vi "CSM - Run Script.vi"(0 "CSM Scripts":string, 1 "Current Module (\"\" to Generate an ID)":string, 7 "Continue If Error? (F)":bool, 9 "Wait (5000ms)":i32=5000, 11 "error in (no error)":errorcluster, 12 "Response Timeout (-2 Using Global Settings)":i32=-2) -> (4 "Response":string[](array[string]), 10 "Scripts Left":string, 15 "error out":errorcluster)   [LabVIEW 2017, in "Communicable State Machine.lvlib"]
doc: "Executes multiple CSM commands in a single batch, supporting synchronous messages, asynchronous messages, and subscriptions.\n\n\n> [!NOTE] <b>CSM Message Target Module Description</b>\n>\n> In Normal Mode, the target module for a CSM message is the specified module name. System-level modules start with a `.` in their name. The target module for a CSM message includes the `.` in the name. For example, if the requested module name is `.System`, the target module for the CSM message is `.System`. In Worker Mode, the target module for a CSM message can only be the overall module name, not the node name. For example, if the requested module name is `Worker#`, the target module for the CSM message is `Worker`. In Chain of Responsibility Mode, the target module for a CSM message can only be the overall module name, not the node name. For example, if the requested module name is `Chain$1`, the target module for the CSM message is `Chain`.\n\n\n-- <b>Controls</b> --\n- <b>Current Module (\"\" to Generate an ID)</b>: Name of the current module. If empty, a temporary ID is generated for debugging purposes to identify the location.\n- <b>CSM Scripts</b>: CSM commands to execute.\n- <b>Continue If Error? (F)</b>: Whether to continue execution if an error occurs. The default is FALSE, which specifies to not continue.\n- <b>Wait (5000 ms)</b>: Timeout duration for waiting. The default is 5000 ms.\n- <b>Response Timeout (-2 Using Global Settings)</b>: Timeout for synchronous calls. The default is -2, which uses the global setting. You can set the global timeout using the CSM - Set TMO of Sync-Reply VI.\n\n-- <b>Indicators</b> --\n- <b>Response</b>: Returned results from executing the script. Only synchronous messages carry returns. The corresponding column for other commands will be an empty string.\n- <b>Scripts Left</b>: Remaining unexecuted scripts."
uses:
  Communicable State Machine.lvlib
  _Shared/CSM Shared.lvlib
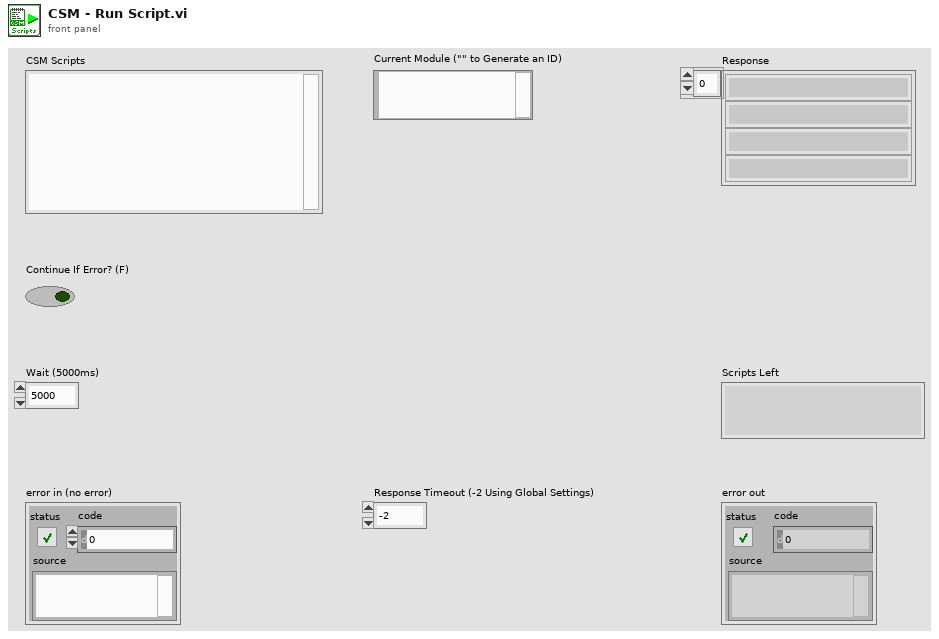
[diagram p1: front panel]
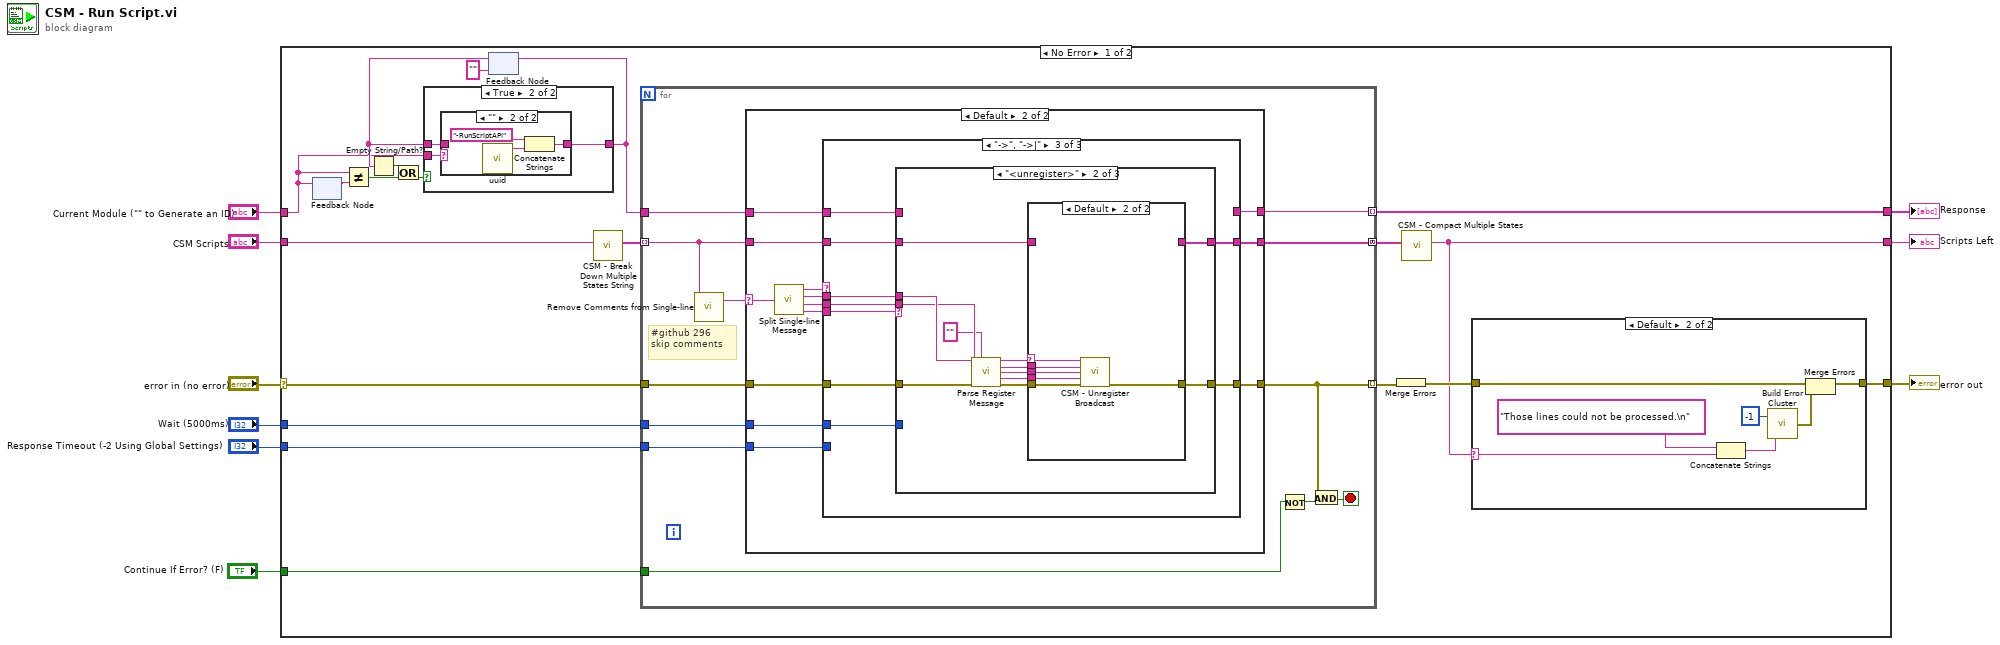
[diagram p0: block diagram]
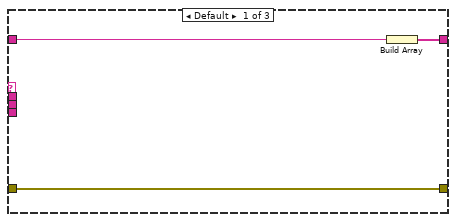
[diagram p6: hidden frame]
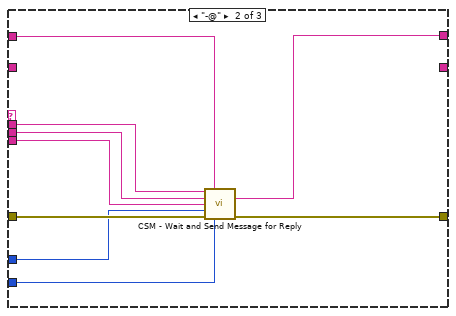
[diagram p7: hidden frame]
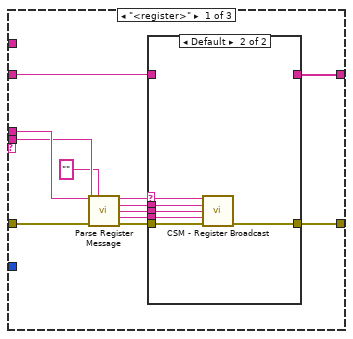
[diagram p8: hidden frame]
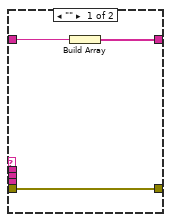
[diagram p9: hidden frame]
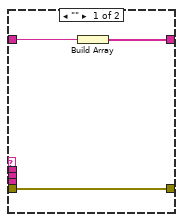
[diagram p10: hidden frame]
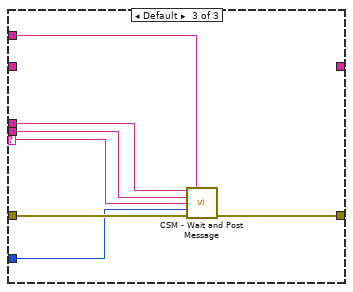
[diagram p11: hidden frame]
diagram:
  n1 = case shown="No Error" "error in (no error)" {
    selector: "error in (no error)" -> [w27 w140]
    tunnel: "CSM Scripts" -> [w26 _]
    tunnel: [w23 _] -> w7
    tunnel: [w22 w140] -> w6
    tunnel: "Current Module (\"\" to Generate an ID)" -> [w11 _]
    tunnel: "Response Timeout (-2 Using Global Settings)" -> [w21 _]
    tunnel: "Wait (5000ms)" -> [w20 _]
    tunnel: "Continue If Error? (F)" -> [w19 _]
    tunnel: [w18 _] -> w1
    frame No Error {
      n2 = feedback #1() -> (w17:string)  [unwired: 1 in]
      n3 = feedback-in #1(w11) -> ()
      n4 = Not Equal?(x=w11, y=w17) -> (x != y?=w16:bool)
      n5 = feedback #2("") -> (w13:string)
      n6 = Empty String/Path?(string/path=w13) -> (empty?=w12:bool)
      n7 = Or(x=w12, y=w16) -> (x .or. y?=w14:bool)
      n8 = case shown="True" w14 {
        tunnel: w13 -> [w30 w33]
        tunnel: w11 -> [_ w32]
        tunnel: [w30 w31] -> w10
        frame False {
        }
        frame True {
          n9 = case shown="\"\"" w32 {
            selector: w32 -> [w34 _]
            tunnel: [w34 w35] -> w31
            tunnel: w33 -> [_ _]
            frame Default {
            }
            frame "" {
              n10 = call "uuid.vi"() -> ("UUID"=w36:string)  [unwired: 11 in]
              n11 = Concatenate Strings("-RunScriptAPI" ("Name (\"\" to Use UUID)"), w36) -> (w35:string)
            }
          }
        }
      }
      n12 = feedback-in #2(w10) -> ()
      n13 = call "CSM - Break Down Multiple States String.vi"("States"=w26) -> ("Multiple States"=w25:string[])  [unwired: 10 in]
      n14 = for {
        tunnel: w25 -> [w54] mode=indexing
        tunnel: w27 -> [w57]
        tunnel: [w49] -> w28 mode=indexing
        tunnel: [w55] -> w24 mode=concatenating
        tunnel: w10 -> [w53]
        tunnel: w21 -> [w52]
        tunnel: w20 -> [w51]
        tunnel: w19 -> [w48]
        tunnel: [w46] -> w18 mode=indexing
        stop <- w50 stop-if-true
        # "#github 296\nskip comments"
        n15 = call "Remove Comments from Single-line.vi"("single-line text"=w54) -> ("single-line text without comments"=w56:string)  [unwired: 2 in]
        n16 = case shown="Default" w56 {
          selector: w56 -> [_ w65]
          tunnel: [w58 w71] -> w49
          tunnel: w57 -> [w58 w70]
          tunnel: [_ w64] -> w55
          tunnel: w54 -> [_ w63]
          tunnel: w53 -> [_ w62]
          tunnel: w52 -> [_ w61]
          tunnel: w51 -> [_ w60]
          tunnel: [_ w59] -> w46
          frame "" {
          }
          frame Default {
            n17 = call "Split Single-line Message.vi"("single-line text"=w65) -> ("operator"=w69:string, "state"=w66:string, "args"=w67:string, "source/target"=w68:string)  [unwired: 6 in]
            n18 = case shown="\"->\", \"->|\"" w69 {
              tunnel: w68 -> [_ w83 w92]
              tunnel: w67 -> [_ w82 w91]
              tunnel: w66 -> [_ w81 w90]
              tunnel: w70 -> [w74 w80 w89]
              tunnel: [w74 w79 w88] -> w71
              tunnel: [w73 _ w87] -> w64
              tunnel: w63 -> [w72 _ w86]
              tunnel: w62 -> [_ w78 w85]
              tunnel: w61 -> [_ w77 _]
              tunnel: w60 -> [_ w76 w84]
              tunnel: [_ w75 _] -> w59
              frame Default {
                n19 = Build Array(w72) -> (w73:string[])
              }
              frame "-@" {
                n20 = call "CSM - Wait and Send Message for Reply.vi"("State"=w81, "Current Module (\"\" to Generate an ID)"=w78, "Arguments (\"\")"=w82, "Target Module"=w83, "Wait (5000ms)"=w76, "Error In (No Error)"=w80, "Response Timeout (-2 Using Global Settings)"=w77) -> ("Response"=w75:string, "error out"=w79:errorcluster)  [unwired: 6 in, 1 out]
              }
              frame "->", "->|" {
                n21 = case shown="\"<unregister>\"" w92 {
                  selector: w92 -> [_ _ w139]
                  tunnel: w91 -> [w98 w118 w138]
                  tunnel: w90 -> [w99 w119 w137]
                  tunnel: w89 -> [w97 w117 w136]
                  tunnel: [w96 w116 w135] -> w88
                  tunnel: [w94 w114 _] -> w87
                  tunnel: w86 -> [w93 w113 _]
                  tunnel: w85 -> [_ _ w134]
                  tunnel: w84 -> [_ _ w133]
                  frame "<register>" {
                    n22 = call "Parse Register Message.vi"("State"=w99, "Module Name"="", "Args"=w98) -> ("Target"=w103:string, "Source"=w102:string, "Status"=w101:string, "Api"=w100:string)  [unwired: 8 in, 1 out]
                    n23 = case shown="Default" w103 {
                      selector: w103 -> [_ w112]
                      tunnel: w102 -> [_ w111]
                      tunnel: w101 -> [_ w110]
                      tunnel: w100 -> [_ w109]
                      tunnel: w97 -> [w106 w108]
                      tunnel: [w106 w107] -> w96
                      tunnel: [w104 _] -> w94
                      tunnel: w93 -> [w105 _]
                      frame "" {
                        n24 = Build Array(w105) -> (w104:string[])
                      }
                      frame Default {
                        n25 = call "CSM - Register Broadcast.vi"("CSM Name(Empty for Broadcast Event)"=w112, "Source CSM Name (* as Default)"=w111, "Trigger"=w110, "API (If \"\", Same as Trigger)"=w109, "Error In"=w108) -> ("error out"=w107:errorcluster)  [unwired: 9 in, 1 out]
                      }
                    }
                  }
                  frame "<unregister>" {
                    n26 = call "Parse Register Message.vi"("State"=w119, "Module Name"="", "Args"=w118) -> ("Target"=w123:string, "Source"=w122:string, "Status"=w121:string, "Api"=w120:string)  [unwired: 8 in, 1 out]
                    n27 = case shown="Default" w123 {
                      selector: w123 -> [_ w132]
                      tunnel: w122 -> [_ w131]
                      tunnel: w121 -> [_ w130]
                      tunnel: w120 -> [_ w129]
                      tunnel: w117 -> [w126 w128]
                      tunnel: [w126 w127] -> w116
                      tunnel: [w124 _] -> w114
                      tunnel: w113 -> [w125 _]
                      frame "" {
                        n28 = Build Array(w125) -> (w124:string[])
                      }
                      frame Default {
                        n29 = call "CSM - Unregister Broadcast.vi"("CSM Name(Empty for Broadcast Event)"=w132, "Source CSM Name (* as Default)"=w131, "Trigger"=w130, "API (\"*\" as Default)"=w129, "Error In"=w128) -> ("error out"=w127:errorcluster)  [unwired: 9 in, 1 out]
                      }
                    }
                  }
                  frame Default {
                    n30 = call "CSM - Wait and Post Message.vi"("State"=w137, "Current Module (\"\" to Generate an ID)"=w134, "Arguments (\"\")"=w138, "Target Module"=w139, "Wait (5000ms)"=w133, "Error In (No Error)"=w136) -> ("error out"=w135:errorcluster)  [unwired: 9 in]
                  }
                }
              }
            }
          }
        }
        n31 = Not(x=w48) -> (.not. x?=w47:bool)
        n32 = And(x=w49, y=w47) -> (x .and. y?=w50:bool)
      }
      n33 = Merge Errors(w28) -> (w29:errorcluster)
      n34 = call "CSM - Compact Multiple States.vi"("Multiple States"=w24) -> ("States"=w23:string)  [unwired: 9 in]
      n35 = case shown="Default" w23 {
        selector: w23 -> [_ w41]
        tunnel: w29 -> [w38 w45]
        tunnel: [w38 w40] -> w22
        frame "" {
        }
        frame Default {
          n36 = Concatenate Strings("Those lines could not be processed.\n" ("String to Prepend to source (\"\")"), w41) -> (w42:string)
          n37 = call "Build Error Cluster.vi"("String to Prepend to Source (\"\")"=w42, "Code"=-1 ("code")) -> ("error out"=w39:errorcluster)
          n38 = Merge Errors(w45, w39) -> (w40:errorcluster)
        }
      }
    }
    frame Error {
    }
  }
  "error out" <- w6
  "Scripts Left" <- w7
  "Response" <- w1
